vi "aim1553sandbox.vi"() -> ()   [LabVIEW 2020]
uses:
  Source/Libraries/Aim_1553_Parameter_ni/_tyedefs/message_type.ctl
  Source/Libraries/Aim_1553_Parameter_ni/_tyedefs/messageAddress_type.ctl
  Source/Libraries/Aim_1553_Parameter_ni/_tyedefs/parameter_type.ctl
  C:/Users/Administrator/Desktop/GIT/Ballard-Arinc-429-XML-Generator/Source/Assemblies/Aim_1553_Parameter_ni/bin/Debug/AIM_1553_Parameter_ni.dll
  Source/Assemblies/Aim_1553_Parameter_ni/bin/Debug/AIM_1553_Parameter_ni.dll
  Source/Libraries/Aim_1553_Parameter_ni/AIM_1553_Parameter_ni.lvlib
panel:
  in  "new parameter file":refnum<k24>
  in  "parameter configuration":T1={"defaultValue"=0.0, "encoding"=0, "name"="param1", "numberOfBits"=31, "offset"=0.0, "scale"=1.0, "signed"=TRUE, "startBit"=0, "unit"="pascal"} {"encoding" items=["BNR", "BCD", "Discrete"]}
  in  "messageAddresses":T2[](array[typedef])=[{"direction"=1, "subAddress"=2, "terminalAddress"=1}] {"direction" items=["Rx", "Tx"]}
  in  "message configuration":T3={"name"="BC to RT1 (SA2)", "numberOfWords"=1, "modeCode"=0, "messageType"=0, "createTimestampChannel"=TRUE, "modeCodeSpecified"=FALSE} {"messageType" items=["BCtoRT", "RTtoBC", "RTtoRT", "MC"]}
  in  "minorFramePeriod":i32=1000
  in  "minor frame name":string="MinorFrame1"
  in  "major frame nme":string="MajorFrame1"
  in  "terminal name":string="BC"
  in  "terminalAddress":i32
  in  "hardwareChannel":i32
  in  "XML path":path=path "C:/Users/Administrator/Desktop/GIT/Ballard-Arinc-429-XML-Generator/Database Examples/ParametersAIM_1553.xml"
  out "error out":errorcluster
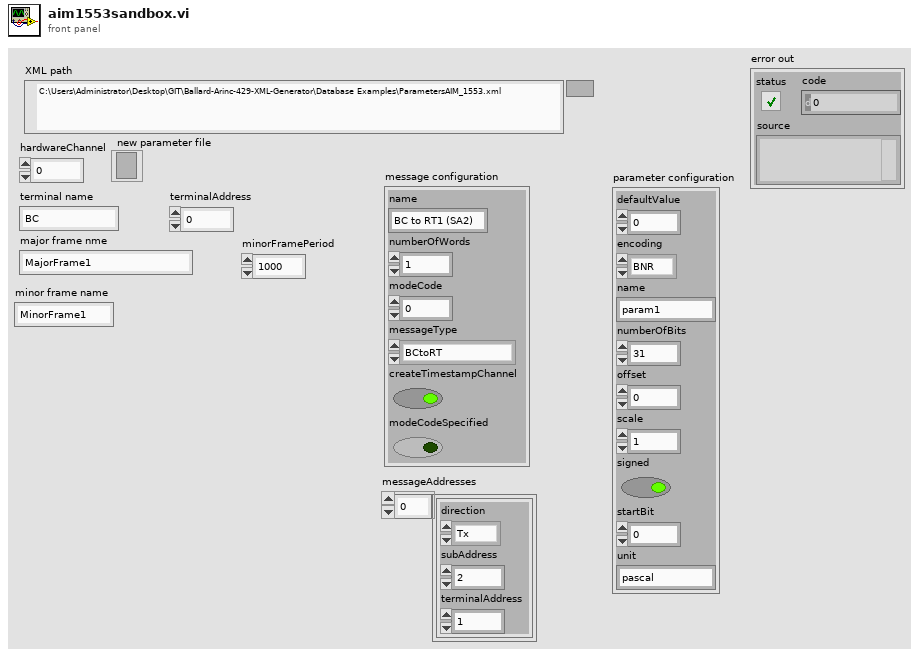
[diagram p1: front panel]
types:
  T1 = typedef "AIM_1553_Parameter_ni.lvlib/parameter_type.ctl" = cluster{"defaultValue":dbl, "encoding":i32, "name":string, "numberOfBits":i32, "offset":dbl, "scale":dbl, "signed":bool, "startBit":i32, "unit":string}
  T2 = typedef "AIM_1553_Parameter_ni.lvlib/messageAddress_type.ctl" = cluster{"direction":i32, "subAddress":i32, "terminalAddress":i32}
  T3 = typedef "AIM_1553_Parameter_ni.lvlib/message_type.ctl" = cluster{"name":string, "numberOfWords":i32, "modeCode":i32, "messageType":i32, "createTimestampChannel":bool, "modeCodeSpecified":bool}
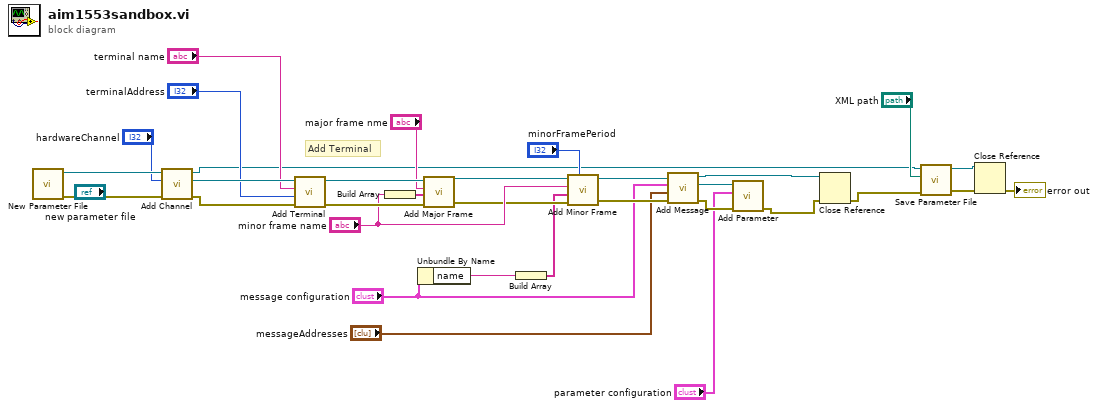
[diagram p0: block diagram]
diagram:
  # "Add Terminal"
  n1 = call "New Parameter File.vi"() -> ("error out"=w26:errorcluster, "new parameter file"=w28:refnum<k24>)  [unwired: 10 in]
  n2 = call "Add Channel.vi"("error in"=w26, "hardwareChannel"="hardwareChannel", "parameter file in"=w28) -> ("error out"=w24:errorcluster, "new channel"=w25:refnum<k24>, "parameter file out"=w2:refnum<k24>)  [unwired: 6 in]
  n3 = call "Add Terminal.vi"("error in"=w24, "terminalAddress"="terminalAddress", "name"="terminal name", "channel in"=w25) -> ("error out"=w22:errorcluster, "channel out"=w23:refnum<k24>)  [unwired: 5 in, 1 out]
  n4 = Build Array("minor frame name") -> (w16:string[])
  n5 = Unbundle By Name("message configuration") -> ("name"=w10:string)
  n6 = call "Add Major Frame.vi"("error in"=w22, "minorFrames"=w16, "name"="major frame nme", "channel in"=w23) -> ("error out"=w17:errorcluster, "channel out"=w15:refnum<k24>)  [unwired: 5 in, 1 out]
  n7 = Build Array(w10) -> (w9:string[])
  n8 = call "Add Minor Frame.vi"("minorFramePeriod"="minorFramePeriod", "error in"=w17, "messageRefs"=w9, "name"="minor frame name", "channel in"=w15) -> ("error out"=w12:errorcluster, "channel out"=w14:refnum<k24>)  [unwired: 4 in, 1 out]
  n9 = call "Add Message.vi"("error in"=w12, "messageAddresses"="messageAddresses", "message configuration"="message configuration", "channel in"=w14) -> ("error out"=w6:errorcluster, "new message"=w7:refnum<k24>, "channel out"=w5:refnum<k24>)  [unwired: 5 in]
  n10 = call "Add Parameter.vi"("error in"=w6, "parameter configuration"="parameter configuration", "message in"=w7) -> ("error out"=w4:errorcluster)  [unwired: 6 in, 2 out]
  n11 = Close Reference(reference=w5, error in (no error)=w4) -> (error out=w3:errorcluster)
  n12 = call "Save Parameter File.vi"("error in"=w3, "XML path"="XML path", "parameter file in"=w2) -> ("error out"=w31:errorcluster, "parameter file out"=w32:refnum<k24>)  [unwired: 6 in, 1 out]
  n13 = Close Reference(reference=w32, error in (no error)=w31) -> (error out=→"error out":errorcluster)
